vi "GetParam.vi"(8 "error in (no error)":errorcluster caption="entrée d'erreur (pas d'erreur)", 11 "California_housing.lvclass":refnum<class "California_housing.lvclass">) -> (0 "error out":errorcluster caption="sortie d'erreur", 2 "fetch_california_housing":T1={"download_if_missing"=TRUE, "Returns"="Data"}, 3 "California_housing.lvclass":refnum<class "California_housing.lvclass">)   [LabVIEW 2020, in "California_housing.lvclass"]
doc: "Get parameters"
uses:
  California_housing.lvclass
  California_housing.lvclass/California_housing.ctl
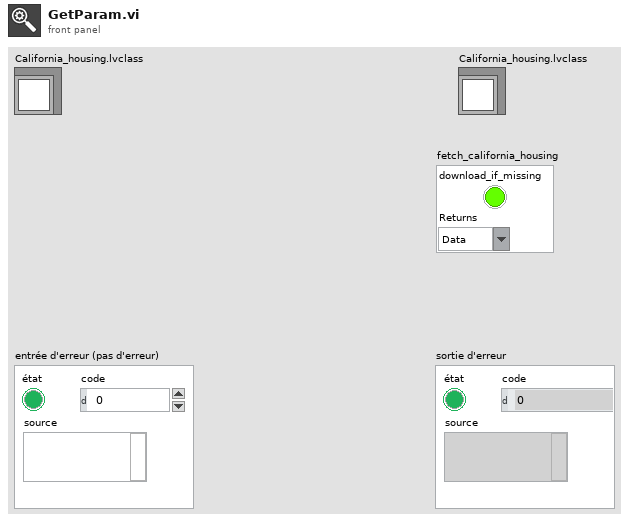
[diagram p1: front panel]
types:
  T1 = cluster{"download_if_missing":bool, "Returns":string}
  T2 = cluster{" download_if_missing ":bool, "Returns":string}
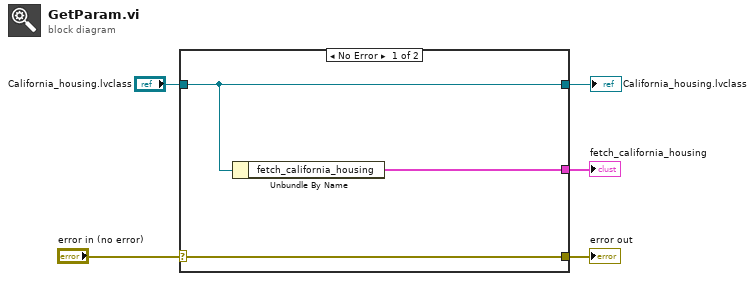
[diagram p0: block diagram]
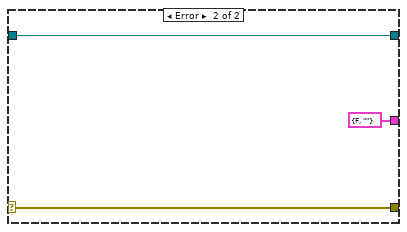
[diagram p2: hidden frame]
diagram:
  n1 = case shown="No Error" "error in (no error)" {
    selector: "error in (no error)" -> [w8 w10]
    tunnel: [w8 w10] -> w4
    tunnel: [w7 w11] -> w1
    tunnel: "California_housing.lvclass" -> [w7 w11]
    tunnel: [w6 T2 {" download_if_missing "=FALSE, "Returns"=""} ("fetch_california_housing")] -> w3
    frame No Error {
      n2 = Unbundle By Name(w7) -> ("fetch_california_housing"=w6:T2)
    }
    frame Error {
    }
  }
  "error out" <- w4
  "fetch_california_housing" <- w3
  "California_housing.lvclass" <- w1
